vi "nirviRandomDataFpgaMultiElementTemplate.vi"(0 "Element in":variant, 1 "Timeout (ms)":i32, 3 "Fifo":T2={"displayName"="", "hardwareName"="", "dataType"=enum."I16", "elementTypeDescriptor"=variant, "terminalTypeDescriptor"=variant, "requestedNumberOfElements"=2, "memoryType"=enum."Look-Up Table", "arbitrationForInterfaceA"=enum."Arbitrate if Multiple Requestors Only", "numberOfElementsPerRead"=1, "arbitrationForInterfaceB"=enum."Always Arbitrate", "numberOfElementsPerWrite"=1, "VI_Defined"=FALSE, "type"=enum."Target-Scoped", "initializationParameters"={"initialized"=FALSE, "VI_Path"=path "", "initialData"=variant}, "disableOnOverflow/Underflow"=FALSE, "interfaceConfiguration"=enum."Read A-Write B", "controlLogic"=enum."Slice Fabric", "actualNumberOfElements"=1027, "dramSelection"="", "dramMaxOustandingRequests"=0, "dramIncludeByteEnables"=FALSE, "dramGrantTime"=0, "fullEmulation"=FALSE, "memoryInMultipleClockDomains"=FALSE, "memoryLatency"=1} {"memoryLatency" items=["0", "1", "2", "3"]}, 4 "Method":T1, 5 "error in (no error)":errorcluster, 6 "Terminal Type Descriptor":variant, 8 "In SCTL":bool, 9 "Input Valid?":bool, 10 "Element Datatype":i32, 11 "Ready for Output?":bool) -> (14 "element":variant, 15 "Timed out":bool, 16 "Ready for Input":bool, 17 "count":u32, 18 "Output Valid":bool, 19 "error out":errorcluster)   [LabVIEW 2017]
uses:
  <vilib>/rvi/DataTransferAndStorage/Container/Common/niFpgaContainerState.ctl
  <vilib>/rvi/DataTransferAndStorage/Container/Common/niFpgaDataTypeControl.ctl
  <vilib>/rvi/DataTransferAndStorage/Container/Common/niFpgaContainerImplementationControl.ctl
  <vilib>/rvi/DataTransferAndStorage/Container/Common/niFpgaContainerArbitrationOptionsControl.ctl
  <vilib>/rvi/DataTransferAndStorage/Container/Common/niFpgaTransferTypeControl.ctl
  <vilib>/rvi/DataTransferAndStorage/Container/Common/niFpgaContainerInitializationParameters.ctl
  <vilib>/rvi/Memory/Memory_Types/niFpgaMemoryInterfaceConfiguration.ctl
  <vilib>/rvi/FIFO/Fifo_Types/niFpgaFifoControlLogicControl.ctl
  <vilib>/rvi/DataTransferAndStorage/Container/Common/niFpgaContainerMemoryLatencyControl.ctl
  <vilib>/rvi/DataTransferAndStorage/Container/Common/niFpgaContainerMethod.ctl
  <instcachedir>/0/nirviRandomDataMultiElementFPGAFIFO_6740B454F3C245F78F76ED91F73FD8DB.lvgen/nirviRandomDataMultiElementFPGAFIFO_6740B454F3C245F78F76ED91F73FD8DB_000.vi
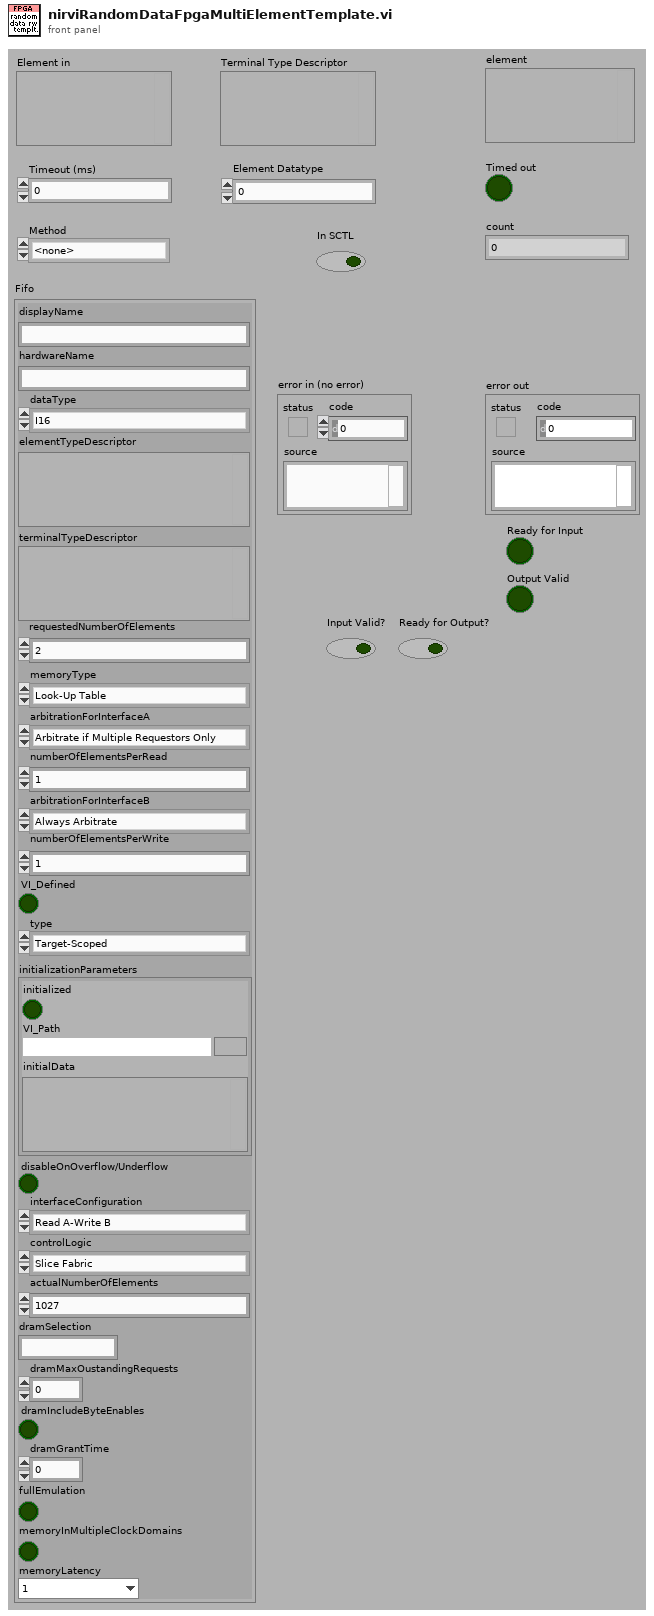
[diagram p1: front panel]
types:
  T1 = typedef "niFpgaContainerMethod.ctl" = enum16{"<none>", "write", "read", "clear", "getNumberOfElementsToWrite", "getNumberOfElementsToRead", "enable", "disable", "flushAndDisable", "getStreamState", "readA", "readB", "dramWrite", "dramWriteWithByteEnables", "dramRequestData", "dramRetrieveData", "readWithoutAcknowledge", "acknowledge", "writeUsingHandshaking", "readUsingHandshaking", "flush"}
  T2 = typedef "niFpgaContainerState.ctl" = cluster{"displayName":string, "hardwareName":string, "dataType":T3, "elementTypeDescriptor":variant, "terminalTypeDescriptor":variant, "requestedNumberOfElements":u32, "memoryType":T4, "arbitrationForInterfaceA":T5, "numberOfElementsPerRead":u32, "arbitrationForInterfaceB":T5, "numberOfElementsPerWrite":u32, "VI_Defined":bool, "type":T6, "initializationParameters":T7, "disableOnOverflow/Underflow":bool, "interfaceConfiguration":T8, "controlLogic":T9, "actualNumberOfElements":u32, "dramSelection":string, "dramMaxOustandingRequests":i32, "dramIncludeByteEnables":bool, "dramGrantTime":u32, "fullEmulation":bool, "memoryInMultipleClockDomains":bool, "memoryLatency":T10}
  T3 = typedef "niFpgaDataTypeControl.ctl" = enum32{"Boolean", "I8", "I16", "I32", "I64", "U8", "U16", "U32", "U64", "FXP", "CustomControl", "SGL"}
  T4 = typedef "niFpgaContainerImplementationControl.ctl" = enum16{"Flip-Flops", "Look-Up Table", "Block Memory", "DRAM"}
  T5 = typedef "niFpgaContainerArbitrationOptionsControl.ctl" = enum16{"Always Arbitrate", "Arbitrate if Multiple Requestors Only", "Never Arbitrate"}
  T6 = typedef "niFpgaTransferTypeControl.ctl" = enum16{"Target-Scoped", "Host to Target - DMA", "Target to Host - DMA", "Peer to Peer Reader", "Peer to Peer Writer", "Bidirectional"}
  T7 = typedef "niFpgaContainerInitializationParameters.ctl" = cluster{"initialized":bool, "VI_Path":path, "initialData":variant}
  T8 = typedef "niFpgaMemoryInterfaceConfiguration.ctl" = enum16{"Read A-Write B", "Read A-Read B"}
  T9 = typedef "niFpgaFifoControlLogicControl.ctl" = enum16{"Slice Fabric", "Target Optimal", "Built-in"}
  T10 = typedef "niFpgaContainerMemoryLatencyControl.ctl" = u16
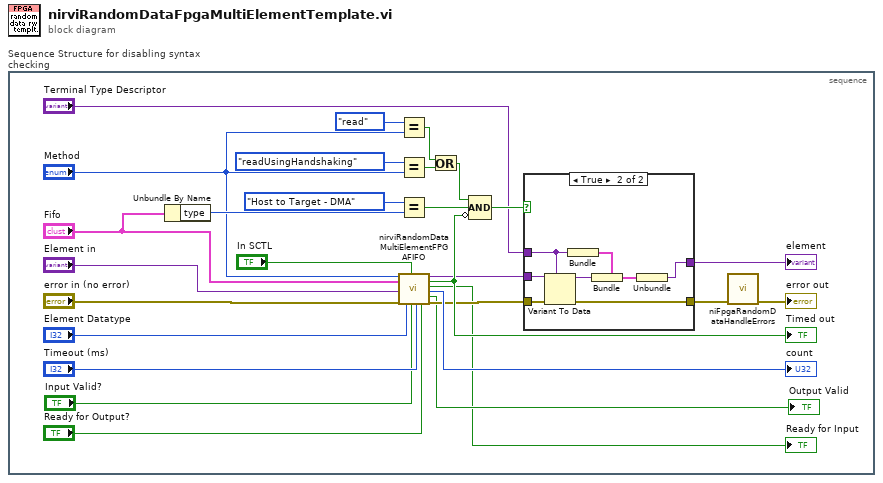
[diagram p0: block diagram]
diagram:
  n1 = stacked-sequence "Sequence Structure for disabling syntax checking" {
    frame #0 {
      n2 = Unbundle By Name("Fifo") -> ("type"=w24:T6)
      n3 = Equal?(x=niFpgaContainerMethod."read", y="Method") -> (x = y?=w2:bool)
      n4 = Equal?(x=niFpgaContainerMethod."readUsingHandshaking", y="Method") -> (x = y?=w3:bool)
      n5 = Equal?(x=niFpgaTransferTypeControl."Host to Target - DMA" ("y"), y=w24) -> (x = y?=w18:bool)
      n6 = call-generic <vilib>:"nirviRandomDataMultiElementFPGAFIFO.vi"("Method"="Method", "Fifo"="Fifo", "element in"="Element in", "error in (no error)"="error in (no error)", "Element Datatype"="Element Datatype", "In SCTL"="In SCTL", "Input Valid?"="Input Valid?", "Timeout (ms)"="Timeout (ms)", "Ready for Output?"="Ready for Output?") -> ("element out"=w13:variant, "Timed out"=w21:bool, "Ready for Input"=→"Ready for Input":bool, "count"=→"count":u32, "Output Valid"=→"Output Valid":bool, "error out"=w16:errorcluster)  [unwired: 5 in]
      "Timed out" <- w21
      n7 = Or(x=w2, y=w3) -> (x .or. y?=w1:bool)
      n8 = Compound Arithmetic op=AND(w1, w18, invert w21) -> (w15:bool)
      n9 = case shown="True" w15 {
        tunnel: w16 -> [w29 w37]
        tunnel: "Terminal Type Descriptor" -> [_ w35]
        tunnel: w13 -> [_ w36]
        tunnel: [w29 w30] -> w11
        tunnel: [_ w31] -> w12
        frame False {
        }
        frame True {
          n10 = Variant To Data(error in=w37, type=w35, Variant=w36) -> (data=w33:variant, error out=w30:errorcluster)
          n11 = Bundle("Terminal Type Descriptor"=w35) -> (w34:cluster{"Terminal Type Descriptor":variant})  [unwired: 1 in]
          n12 = Bundle(cluster=w34, "Terminal Type Descriptor"=w33) -> (w32:cluster{"Terminal Type Descriptor":variant})
          n13 = Unbundle(w32) -> ("Terminal Type Descriptor"=w31:variant)
        }
      }
      "element" <- w12
      n14 = call <vilib>:"niFpgaRandomDataHandleErrors.vi"("error in"=w11) -> ("error out"=→"error out":errorcluster)  [unwired: 14 out]
    }
  }
